vi "CalculoOndaContinua.vi"(0 "OndaIn":cluster{"X":dbl, "Y":dbl}[](array[cluster]), 1 "PicoMax":dbl) -> (7 "OndaOut":cluster{"X":dbl, "Y":dbl}[](graph))   [LabVIEW 2019]
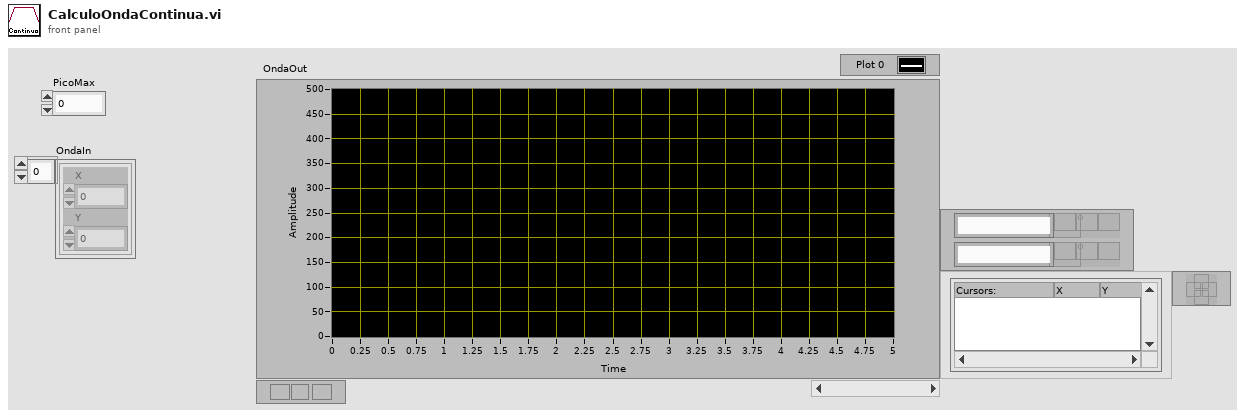
[diagram p1: front panel]
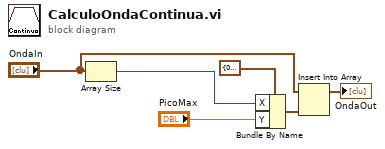
[diagram p0: block diagram]
diagram:
  n1 = Array Size(array="OndaIn") -> (size(s)=w1:i32)
  n2 = Bundle By Name(cluster=cluster{"X":dbl, "Y":dbl} {"X"=0.0, "Y"=0.0} ("new element/subarray"), "X"=w1, "Y"="PicoMax") -> (w3:cluster{"X":dbl, "Y":dbl})
  n3 = Insert Into Array(array="OndaIn", new element=w3) -> (→"OndaOut":cluster{"X":dbl, "Y":dbl}[])  [unwired: 1 in]
